vi "_PC_Pub_FM reset.vi"(8 "error in (no error)":errorcluster, 11 "FM in":refnum<class "FM.lvclass">) -> (0 "error out":errorcluster, 3 "FM out":refnum<class "FM.lvclass">)   [LabVIEW 2018, in "FM.lvclass"]
uses:
  FM.lvclass
  ctl/_PC_Pub_FM fileReadFuncEnum.ctl
  FM.lvclass/FM.ctl
  TDMSAdv.lvclass
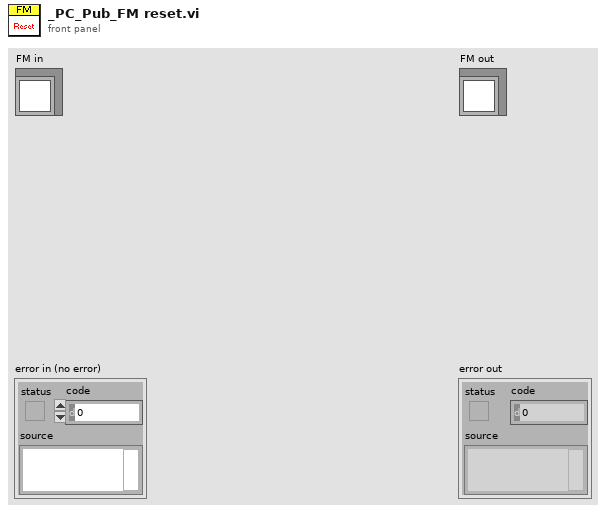
[diagram p1: front panel]
types:
  T1 = typedef "_PC_Pub_FM fileReadFuncEnum.ctl" = enum16{"getAllInfo", "getChromatogram", "getDataItems", "getTimeStamp", "getIdxData", "getIonization", "getRemark", "getAttrFormat"}
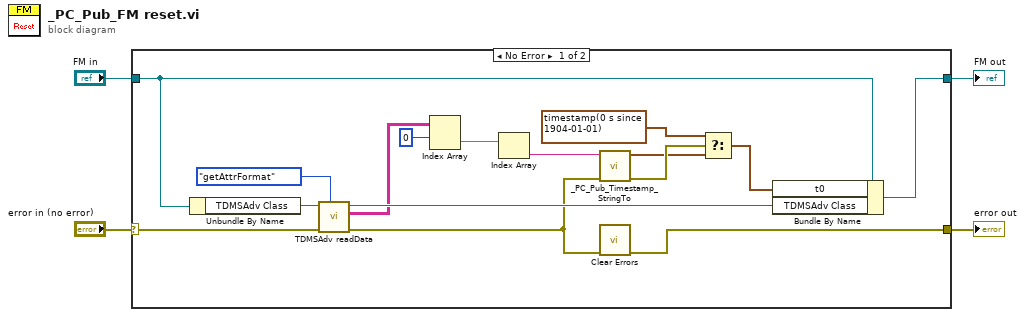
[diagram p0: block diagram]
diagram:
  n1 = case shown="No Error" "error in (no error)" {
    selector: "error in (no error)" -> [w18 w22]
    tunnel: [w16 w22] -> w3
    tunnel: [w20 w21] -> w1
    tunnel: "FM in" -> [w19 w21]
    frame No Error {
      n2 = Unbundle By Name(w19) -> ("TDMSAdv Class"=w17:refnum<class "TDMSAdv.lvclass">)
      n3 = call "TDMSAdv readData.vi"("readEvent"=_PC_Pub_FM_fileReadFuncEnum."getAttrFormat", "error in (no error)"=w18, "TDMSAdv in"=w17) -> ("error out"=w7:errorcluster, "outputArr"=w5:string[][], "TDMSAdv out"=w14:refnum<class "TDMSAdv.lvclass">)  [unwired: 5 in, 1 out]
      n4 = Index Array(array=w5, index (row)=0) -> (element=w11:string[])  [unwired: 1 in]
      n5 = Index Array(array=w11) -> (element=w12:string)  [unwired: 1 in]
      n6 = call "_PC_Pub_Timestamp_StringTo.vi"("error in"=w7, "Timestring"=w12) -> ("error out"=w10:errorcluster, "Timestamp"=w9:timestamp)  [unwired: 8 in]
      n7 = call <vilib>:"Clear Errors.vi"("error in (no error)"=w7) -> ("error out"=w16:errorcluster)  [unwired: 5 in, 1 out]
      n8 = Select(t=timestamp(0 s since 1904-01-01), s=w10, f=w9) -> (s? t:f=w15:timestamp)
      n9 = Bundle By Name(cluster=w19, "t0"=w15, "TDMSAdv Class"=w14) -> (w20:refnum<class "FM.lvclass">)
    }
    frame Error {
    }
  }
  "error out" <- w3
  "FM out" <- w1
